vi "Read Parameters from Last Call.vi"(8 "error in (no error)":errorcluster, 11 "LabSpy in":refnum<class "LabSpy.lvclass">) -> (0 "error out":errorcluster, 2 "Last Call Parameters":variant, 3 "LabSpy out":refnum<class "LabSpy.lvclass">)   [LabVIEW 2013, in "LabSpy.lvclass"]
doc: "Get the parameters from the final call of the spy."
uses:
  LabSpy.lvclass
  LabSpy.lvclass/LabSpy.ctl
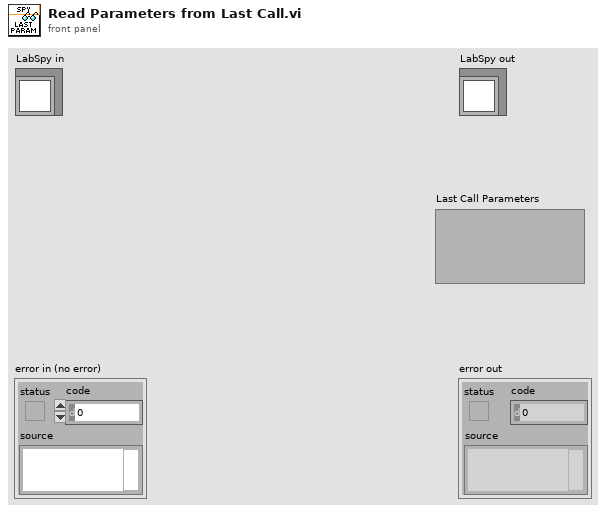
[diagram p1: front panel]
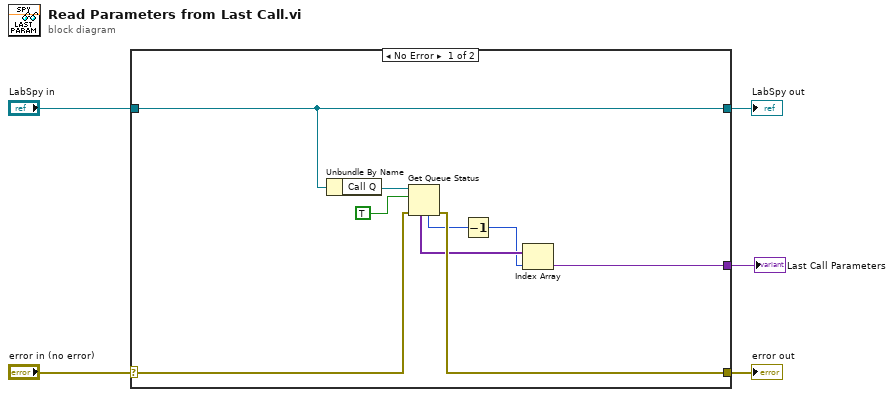
[diagram p0: block diagram]
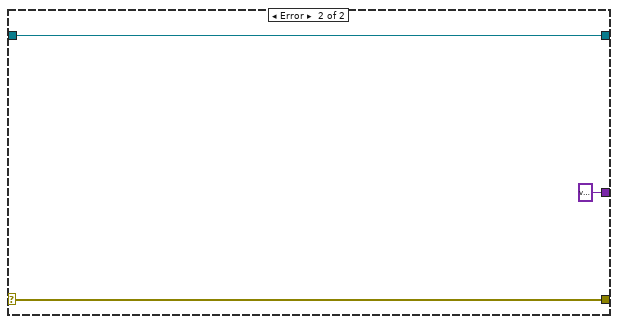
[diagram p2: hidden frame]
diagram:
  n1 = case shown="No Error" "error in (no error)" {
    selector: "error in (no error)" -> [w11 w17]
    tunnel: [w10 w17] -> w4
    tunnel: [w14 w16] -> w2
    tunnel: "LabSpy in" -> [w14 w16]
    tunnel: [w6 variant ("Variant")] -> w1
    frame No Error {
      n2 = Unbundle By Name(w14) -> ("Call Q"=w13:refnum<queue>)
      n3 = Get Queue Status(queue=w13, return elements? (F)=TRUE, error in (no error)=w11) -> (error out=w10:errorcluster, # elements in queue=w9:i32, elements=w8:variant[])  [unwired: 5 out]
      n4 = Decrement(x=w9) -> (x-1=w7:i32)
      n5 = Index Array(array=w8, index=w7) -> (element=w6:variant)
    }
    frame Error {
    }
  }
  "error out" <- w4
  "LabSpy out" <- w2
  "Last Call Parameters" <- w1
